vi "AddFreeField.vi"(8 "error in (no error)":errorcluster, 10 "Coordinate":cluster{"x":i16, "y":i16}, 11 "SnakeGame in":refnum<class "SnakeGame.lvclass">) -> (0 "error out":errorcluster, 3 "SnakeGame out":refnum<class "SnakeGame.lvclass">)   [LabVIEW 2019, in "RT_Game.lvlib" / "SnakeGame.lvclass"]
uses:
  SnakeGame.lvclass
  SnakeGame.lvclass/SnakeGame.ctl
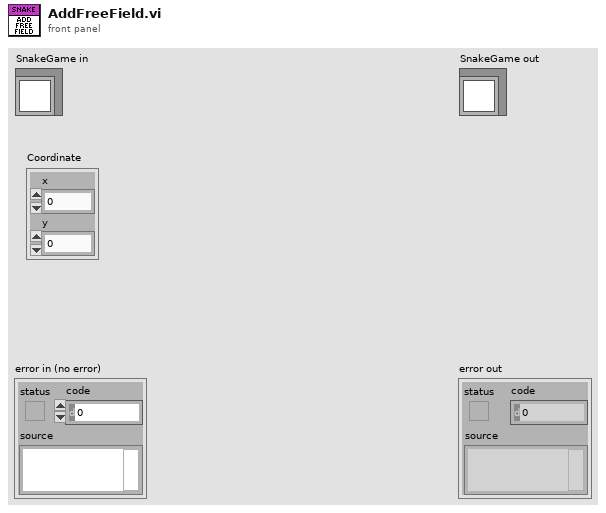
[diagram p1: front panel]
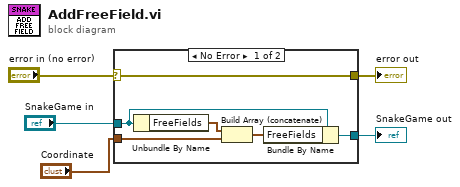
[diagram p0: block diagram]
diagram:
  n1 = case shown="No Error" "error in (no error)" {
    selector: "error in (no error)" -> [w11 w13]
    tunnel: [w11 w13] -> w4
    tunnel: [w10 w12] -> w2
    tunnel: "SnakeGame in" -> [w9 w12]
    tunnel: "Coordinate" -> [w6 _]
    frame No Error {
      n2 = Unbundle By Name(w9) -> ("FreeFields"=w7:cluster{"x":i16, "y":i16}[])
      n3 = Build Array (concatenate)(w7, w6) -> (w8:cluster{"x":i16, "y":i16}[])
      n4 = Bundle By Name(cluster=w9, "FreeFields"=w8) -> (w10:refnum<class "SnakeGame.lvclass">)
    }
    frame Error {
    }
  }
  "error out" <- w4
  "SnakeGame out" <- w2
